vi "HEAD.vi"(6 "timeout":i32=10000, 8 "error in":errorcluster, 10 "url":string, 11 "advanced-http-client in":refnum<class "advanced-http-client.lvclass">) -> (0 "error out":errorcluster, 2 "response out":refnum<class "response.lvclass">, 3 "advanced-http-client out":refnum<class "advanced-http-client.lvclass">)   [LabVIEW 2020, in "advanced-http-client.lvclass"]
uses:
  advanced-http-client.lvclass
  advanced-http-client.lvclass/advanced-http-client.ctl
  <vilib>/NI/Advanced HTTP Client/Session.lvclass
  response/response.lvclass
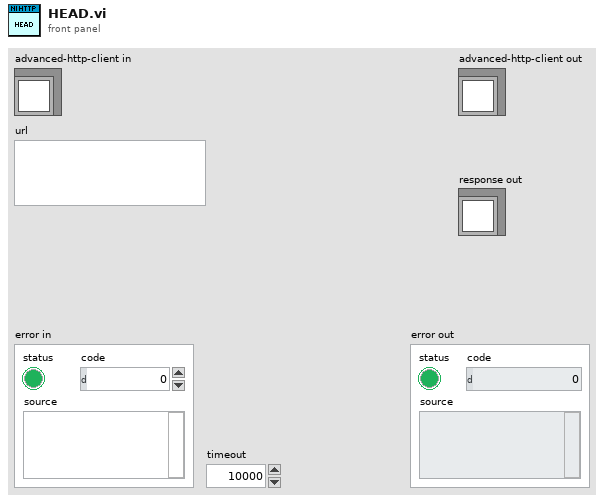
[diagram p1: front panel]
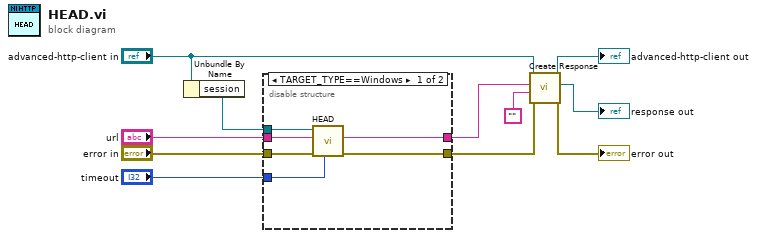
[diagram p0: block diagram]
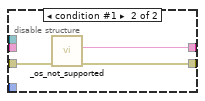
[diagram p2: hidden frame]
diagram:
  n1 = Unbundle By Name("advanced-http-client in") -> ("session"=w8:refnum<class "Session.lvclass">)
  n2 = disable-structure shown="TARGET_TYPE==Windows" {
    disable-tunnel: [w17 w19] -> w3
    disable-tunnel: "error in" -> [w16 w20]
    disable-tunnel: "url" -> [w15 _]
    disable-tunnel: "timeout" -> [w14 _]
    disable-tunnel: w8 -> [w13 _]
    disable-tunnel: [w12 w18] -> w6
    frame condition #0 (active) {
      n3 = call <vilib>:"HEAD.vi"("timeout"=w14, "error in"=w16, "url"=w15, "session in"=w13) -> ("error out"=w17:errorcluster, "headers"=w12:string)  [unwired: 4 in, 2 out]
    }
    frame condition #1 {
      n4 = call "_os_not_supported.vi"("error in (no error)"=w20) -> ("error out"=w19:errorcluster, "headers"=w18:string)  [unwired: 9 in]
    }
  }
  n5 = call-dynamic "Create Response.vi"("error in (no error)"=w3, "body"="", "headers"=w6, "http-client"="advanced-http-client in") -> ("error out"=→"error out":errorcluster, "response out"=→"response out":refnum<class "response.lvclass">, "http-client out"=→"advanced-http-client out":refnum<class "advanced-http-client.lvclass">)  [unwired: 5 in]
